vi "Database Check If Table Exit.vi"(8 "error in (no error)":errorcluster, 10 "Table":string="Select * from xx", 11 "Database in":refnum<class "Database.lvclass">) -> (0 "error out":errorcluster, 2 "Exit?":bool, 3 "Database out":refnum<class "Database.lvclass">)   [LabVIEW 2015, in "Database.lvclass"]
uses:
  Database.lvclass
  Database.lvclass/Database.ctl
  <vilib>/addons/database/Connection.llb/DB Tools Open Connec (String).vi
  <vilib>/addons/database/Connection.llb/Conn Execute.vi
  <vilib>/addons/database/Recordset.llb/Rec Destroy - Connection.vi
  <vilib>/addons/database/NI_Database_API.lvlib
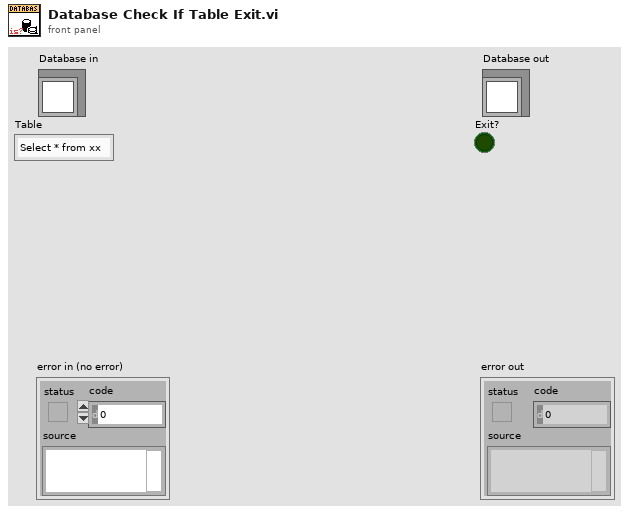
[diagram p1: front panel]
types:
  T1 = typedef "NI_Database_API.lvlib/Conn ObjectReference.ctl" = refnum<k1>
  T2 = typedef "NI_Database_API.lvlib/Rec ObjectReference.ctl" = refnum<k1>
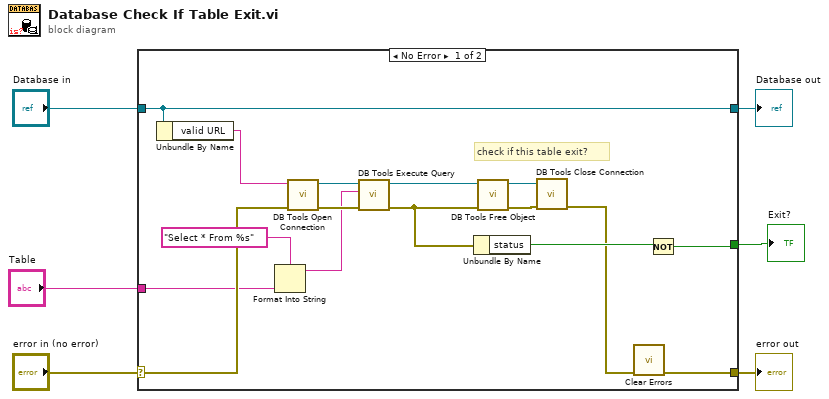
[diagram p0: block diagram]
diagram:
  n1 = case shown="No Error" "error in (no error)" {
    selector: "error in (no error)" -> [w18 w24]
    tunnel: [w7 w24] -> w5
    tunnel: [w22 w23] -> w3
    tunnel: "Database in" -> [w22 w23]
    tunnel: [w9 _] -> w2
    tunnel: "Table" -> [w14 _]
    frame No Error {
      # "check if this table exit?"
      n2 = Unbundle By Name(w22) -> ("valid URL"=w21:string)
      n3 = Format Into String(format string="Select * From %s", w14) -> (resulting string=w12:string)  [unwired: 2 in, 1 out]
      n4 = call-poly <vilib>:"DB Tools Open Connection.vi"("error in (no error)"=w18, "connection information"=w21) -> ("error out"=w19:errorcluster, "connection reference"=w20:T1)  [unwired: 6 in]
      n5 = call-poly <vilib>:"DB Tools Execute Query.vi"("error in (no error)"=w19, "SQL query"=w12, "connection reference"=w20) -> ("error out"=w11:errorcluster, "recordset reference"=w17:T2)  [unwired: 5 in]
      n6 = Unbundle By Name(w11) -> ("status"=w10:bool)
      n7 = call-poly <vilib>:"DB Tools Free Object.vi"("error in (no error)"=w11, "recordset reference"=w17) -> ("error out"=w15:errorcluster, "connection reference"=w16:T1)  [unwired: 8 in]
      n8 = call <vilib>:"DB Tools Close Connection.vi"("error in (no error)"=w15, "connection reference"=w16) -> ("error out"=w8:errorcluster)  [unwired: 5 in]
      n9 = call <vilib>:"Clear Errors.vi"("error in (no error)"=w8) -> ("error out"=w7:errorcluster)  [unwired: 5 in, 1 out]
      n10 = Not(x=w10) -> (.not. x?=w9:bool)
    }
    frame Error {
    }
  }
  "error out" <- w5
  "Database out" <- w3
  "Exit?" <- w2
